vi "vending machine.vi"() -> ()   [LabVIEW 2019]
panel:
  out "money deposited":string
  out "dispensed":bool
  in  "five rupee":bool
  in  "ten rupee":bool
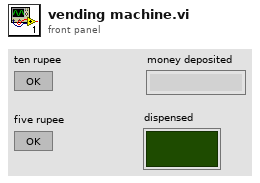
[diagram p1: front panel]
types:
  T1 = enum16{"start", "5 rupee", "ten rupee", "dispensed"}
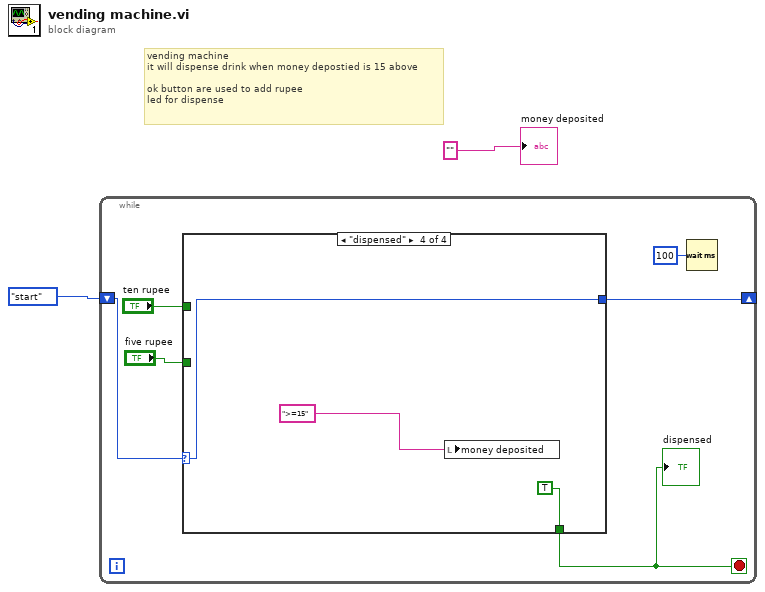
[diagram p0: block diagram]
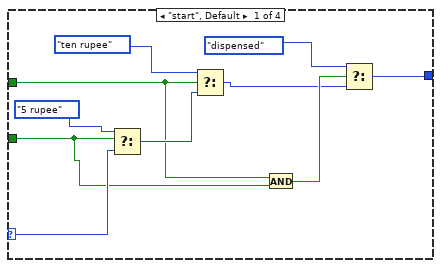
[diagram p2: hidden frame]
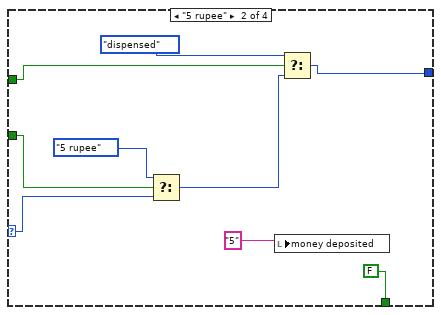
[diagram p3: hidden frame]
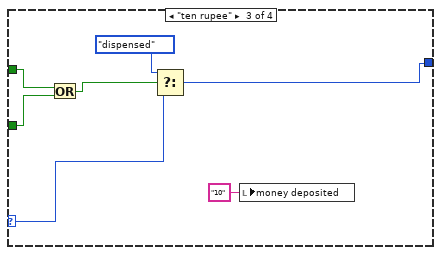
[diagram p4: hidden frame]
diagram:
  # "vending machine \nit will dispense drink when money depostied is 15 above\n\nok button are used to add rupee\nled for dispense"
  n1 = while {
    shift-right: [w5] -> _
    shift-left: T1."start" -> [w8]
    stop <- w4 stop-if-true
    n2 = case shown="\"dispensed\"" w8 {
      selector: w8 -> [w18 w27 w33 w37]
      tunnel: "five rupee" -> [w15 w26 w30 _]
      tunnel: "ten rupee" -> [w16 w25 w31 _]
      tunnel: [w12 w23 w32 w37] -> w5
      tunnel: [_ FALSE _ TRUE] -> w4
      frame "start", Default {
        n3 = Select(t=T1."5 rupee", s=w15, f=w18) -> (s? t:f=w17:T1)
        n4 = Select(t=T1."ten rupee", s=w16, f=w17) -> (s? t:f=w13:T1)
        n5 = And(x=w16, y=w15) -> (x .and. y?=w14:bool)
        n6 = Select(t=T1."dispensed", s=w14, f=w13) -> (s? t:f=w12:T1)
      }
      frame "5 rupee" {
        n7 = Select(t=T1."5 rupee", s=w26, f=w27) -> (s? t:f=w24:T1)
        n8 = local write "money deposited"("5") -> ()
        n9 = Select(t=T1."dispensed", s=w25, f=w24) -> (s? t:f=w23:T1)
      }
      frame "ten rupee" {
        n10 = Or(x=w31, y=w30) -> (x .or. y?=w29:bool)
        n11 = Select(t=T1."dispensed", s=w29, f=w33) -> (s? t:f=w32:T1)
        n12 = local write "money deposited"("10" ("money deposited")) -> ()
      }
      frame "dispensed" {
        n13 = local write "money deposited"(">=15") -> ()
      }
    }
    "dispensed" <- w4
    n14 = Wait (ms)(milliseconds to wait=u32 100) -> ()  [unwired: 1 out]
  }
  "money deposited" <- "" ("money deposited")
